vi "Leaktest DAQ v33w.vi"() -> ()   [LabVIEW 2020]
uses:
  Leaktest Temp Mode Select Enum.ctl
  System Directory Type.ctl
  Cfg Cluster Typedef.ctl
  ULx Create Channel (AI-Temperature).vi
  ULx Create Channel (DO-Digital Output).vi
  ULx Create Channel (DI-Digital Input).vi
  ULx Read (Analog 1D DBL NChan 1Samp).vi
  ULx Write (Digital 1D Bool 1Chan 1Samp).vi
  ULx Read (Digital 1D Bool 1Chan 1Samp).vi
panel:
  in  "USB Temp mS":u32=5
  in  "Fallback Location":T2={"Log directory type"=1, "Rel Log Path"="LeakTestData"} {"Log directory type" items=["User Home"=0, "User Desktop"=1, "User Documents"=2, "User Application Data"=3, "User Preferences"=4, "User Temporary"=5, "Public Documents"=6, "Public Application Data"=7, "Public Preferences"=8, "Public Cache"=13, "System Core Libraries"=9, "System Installed Libraries"=10, "Application Files"=11, "Boot Volume Root"=12]}
  in  "Log Dir Path":path=path "\\\\spa-mu2e-network\\Files/LeakRateRawData"
  out "TP loop mS":u32(slide) scale=0.0..100.0
  in  "Chart Dly mS":u32=10
  out "Max Chart Hrs":dbl
  out "Actual cfg file path":path
  in  "Save Cfg":bool
  out "Config Clst":T3={"Log Dir Path"=path "\\\\spa-mu2e-network\\Files/LeakRateRawData", "File Log Sec"=30.0, "34970A Sec"=1.0, "Chart hrs1"=0.25, "Chart hrs2"=0.25, "Filnen Fmt"="%y%m%d_%H%M_MN#.txt", "Temp chans"="Dev1/Ti0, Dev1/Ti2, Dev1/Ti4", "DI Lines"="Dev1/AuxPort/Di2:3", "DO Lines"="Dev1/AuxPort/Do0:1", "VISA ID 34970A"="34970A", "Baud Rate"=enum."38400", "Time Fmt"=enum."Days"} {"Chart hrs2" format="%.1f"; "Chart hrs1" format="%.1f"; "34970A Sec" format="%.1f"; "File Log Sec" format="%.1f"}
  in  "Cfg Filename":string="Leaktest.ini"
  in  "Cfg File Loc":T4={"Cfg directory type"=3, "Rel Log Path"="LeakTest"} {"Cfg directory type" items=["User Home"=0, "User Desktop"=1, "User Documents"=2, "User Application Data"=3, "User Preferences"=4, "User Temporary"=5, "Public Documents"=6, "Public Application Data"=7, "Public Preferences"=8, "Public Cache"=13, "System Core Libraries"=9, "System Installed Libraries"=10, "Application Files"=11, "Boot Volume Root"=12]}
  in  "Time Fmt":enum16{"H:M:S", "Days", "Secs"}(ring)=enum."Days"
  in  "Filnename Format":string="%y%m%d_%H%M_MN#.txt"
  in  "File Log Sec":u32=30
  in  "Header":string[](array[string])=["Elap days", "Fill PSIA", "Ref PSIA", "Diff \"H2O", "Encl degC", "Room degC", "Heater %"]
  out "Heat Safety 2":bool
  out "Heat Safety 1":bool
  in  "Chart Hrs 2":dbl=0.5 min=0.25 max=24.0 step=0.25
  in  "Chart t0 Hrs 2":dbl min=0.0 max=23.0 step=0.25
  in  "Chart t0 Hrs 1":dbl min=0.0 max=23.0 step=0.25
  in  "Chart Hrs 1":dbl=0.5 min=0.25 max=24.0 step=0.25
  in  "34970A Scan Sec":u32=10
  in  "Pressures":T5
  in  "Press Scaling":T6(array[cluster])=[{"Gain"=5.0, "Offset"=0.0, "Units"="PSI", "Channel"="101", "Name"="Fill 1"}, {"Gain"=7.5, "Offset"=-7.5, "Units"="PSI", "Channel"="102", "Name"="Ref 1"}, {"Gain"=2.0, "Offset"=0.0, "Units"="H2O", "Channel"="103", "Name"="Diff 1"}, {"Gain"=7.5, "Offset"=-7.5, "Units"="PSI", "Channel"="104", "Name"="Fill 2"}, {"Gain"=7.5, "Offset"=-7.46, "Units"="PSI", "Channel"="105", "Name"="Ref 2"}, {"Gain"=2.0, "Offset"=-0.038, "Units"="H2O", "Channel"="106", "Name"="Diff 2"}]
  in  "VISA 34970A":refnum<visa-resource-name>="34970A"
  in  "34970A RS232 Cfg":T7={"Timeout Value (10000)"=2000, "Baud Rate"=enum."38400", "Flow Control (1:XON / XOFF)"=enum."RTS / CTS"}
  out "Diff H2O 2":dbl format="%.3f"
  out "Heat% 2":dbl
  out "Heat% 1":dbl
  out "Heat% Cht 2":dbl(graph)
  out "Heat% Cht 1":dbl(graph)
  in  "DI Lines":refnum<k21>="Dev1/AuxPort/Di2:3"
  in  "DO Lines":refnum<k21>="Dev1/AuxPort/Do0:1"
  in  "Temp input chans":refnum<k21>="Dev1/Ti0, Dev1/Ti2, Dev1/Ti4"
  in  "TP Cycle  mS":dbl=5000.0 min=1000.0 max=30000.0
  in  "TP loop mS":u32=50
  out "Heater Safety":cluster{"Encl 1":bool, "Encl 2":bool}
  in  "Heater Out  T/F":bool[](array[boolean])
  in  "Temp Intvl Sec":u32=1
  in  "output range":cluster{"output high":dbl, "output low":dbl}={"output high"=100.0, "output low"=0.0}
  in  "Control Params":T8={"Setpt C"=24.0, "PID"={" gain (Kc)"=180.0, "integral min"=5.0, "derivative min"=0.0}} {"Setpt C" format="%.2f"; "PID"."derivative min" format="%.3f"; "PID"."integral min" format="%.3f"; "PID"."gain (Kc)" format="%.3f"}
  out "error out":errorcluster
  in  "Manual %":cluster{"Man 1":dbl, "Man 2":dbl} {"Man 2" format="%.1f"; "Man 1" format="%.1f"}
  in  "Control Mode":cluster{"Encl 1":T9, "Encl 2":T9}
  out "Heat%":dbl[](array[numeric]) format="%.2f"
  out "Exit 2":bool
  out "Filename 2":string
  in  "Test stop 2":bool
  out "Run/Stop 2":bool
  in  "Test start 2":bool
  out "Room degC 2":dbl format="%.2f"
  out "Encl degC 2":dbl format="%.2f"
  out "Absolute Pressure Cht 2":cluster{"Fill PSIA 1":dbl, "Fill PSIA 2":dbl}(graph)
  out "Diff Pressure Cht 2":dbl(graph)
  out "Temperature Cht 2":T10(graph)
  out "Ref PSIA 2":dbl format="%.2f"
  out "Fill PSIA 2":dbl format="%.2f"
  out "Filename 1":string
  in  "Test stop 1":bool
  out "Run/Stop 1":bool
  in  "Test start 1":bool
  out "Room degC 1":dbl format="%.2f"
  out "Encl degC 1":dbl format="%.2f"
  out "Absolute Pressure Cht 1":cluster{"Fill PSIA 1":dbl, "Fill PSIA 2":dbl}(graph)
  out "Diff Pressure Cht 1":dbl(graph)
  out "Temperature Cht 1":T10(graph)
  in  "Exit":bool
  out "Ref PSIA 1":dbl format="%.2f"
  out "Diff H2O  1":dbl format="%.3f"
  out "Fill PSIA 1":dbl format="%.2f"
  # "`"
  # "```"
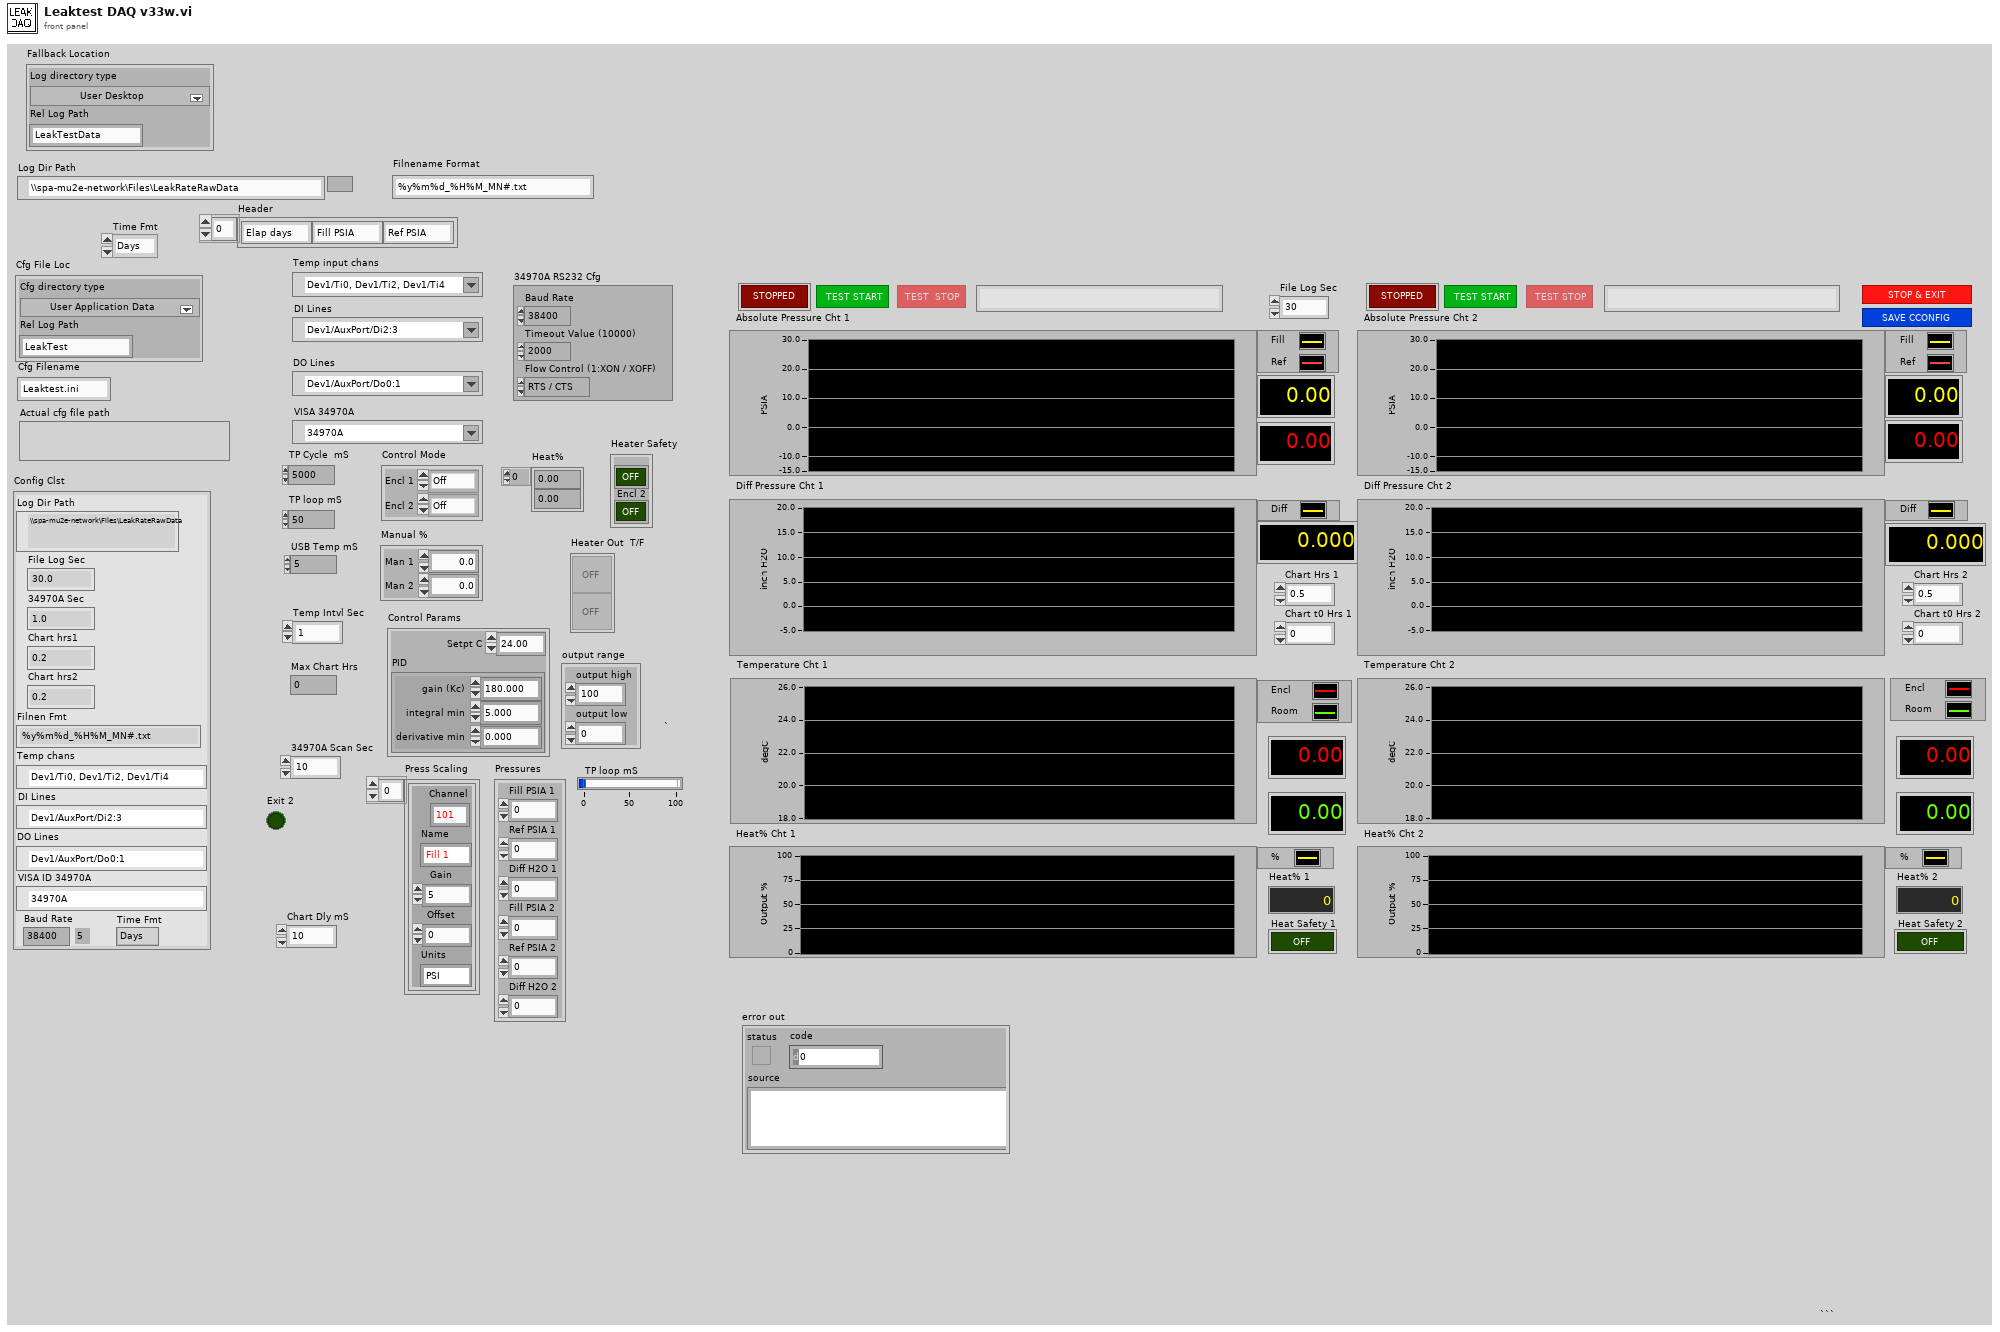
[diagram p1: front panel]
types:
  T1 = typedef "System Directory Type.ctl" = i32
  T2 = cluster{"Log directory type":T1, "Rel Log Path":string}
  T3 = typedef "Cfg Cluster Typedef.ctl" = cluster{"Log Dir Path":path, "File Log Sec":dbl, "34970A Sec":dbl, "Chart hrs1":dbl, "Chart hrs2":dbl, "Filnen Fmt":string, "Temp chans":refnum<k21>, "DI Lines":refnum<k21>, "DO Lines":refnum<k21>, "VISA ID 34970A":refnum<visa-resource-name>, "Baud Rate":enum16{"1200", "2400", "4800", "9600", "19200", "38400", "57600", "115200"}, "Time Fmt":enum16{"H:M:S", "Days", "Secs"}}
  T4 = cluster{"Cfg directory type":T1, "Rel Log Path":string}
  T5 = cluster{"Fill PSIA 1":dbl, "Ref PSIA 1":dbl, "Diff H2O 1":dbl, "Fill PSIA 2":dbl, "Ref PSIA 2":dbl, "Diff H2O 2":dbl}
  T6 = cluster{"Gain":dbl, "Offset":dbl, "Units":string, "Channel":string, "Name":string}[]
  T7 = cluster{"Timeout Value (10000)":u32, "Baud Rate":enum16{"1200", "2400", "4800", "9600", "19200", "38400", "57600", "115200"}, "Flow Control (1:XON / XOFF)":enum16{"None", "XON / XOFF", "RTS / CTS", "DTR / DSR"}}
  T8 = cluster{"Setpt C":dbl, "PID":cluster{" gain (Kc)":dbl, "integral min":dbl, "derivative min":dbl}}
  T9 = typedef "Leaktest Temp Mode Select Enum.ctl" = enum16{"Off", "Manual", "Auto"}
  T10 = cluster{"Temperature 7":dbl, "Temperature 8":dbl}
  T11 = enum16{"Remote Trigger", "Immediate Trigger", "Wait for Trigger", "Abort Scan"}
  T12 = enum8{"Enabled", "Disabled", "Disabled and Grayed Out"}
  T13 = enum16{"1200", "2400", "4800", "9600", "19200", "38400", "57600", "115200"}
  T14 = cluster{"data[0]":dbl, "data[1]":dbl, "data[2]":dbl}
  T15 = cluster{"Fill PSIA 1":dbl, "Ref PSIA 1":dbl, "Diff H2O  1":dbl, "Encl degC 1":dbl, "Room degC 1":dbl, "Heat% 1":dbl}
  T16 = cluster{"Fill PSIA 2":dbl, "Ref PSIA 2":dbl, "Diff H2O 2":dbl, "Encl degC 2":dbl, "Room degC 2":dbl, "Heat% 2":dbl}
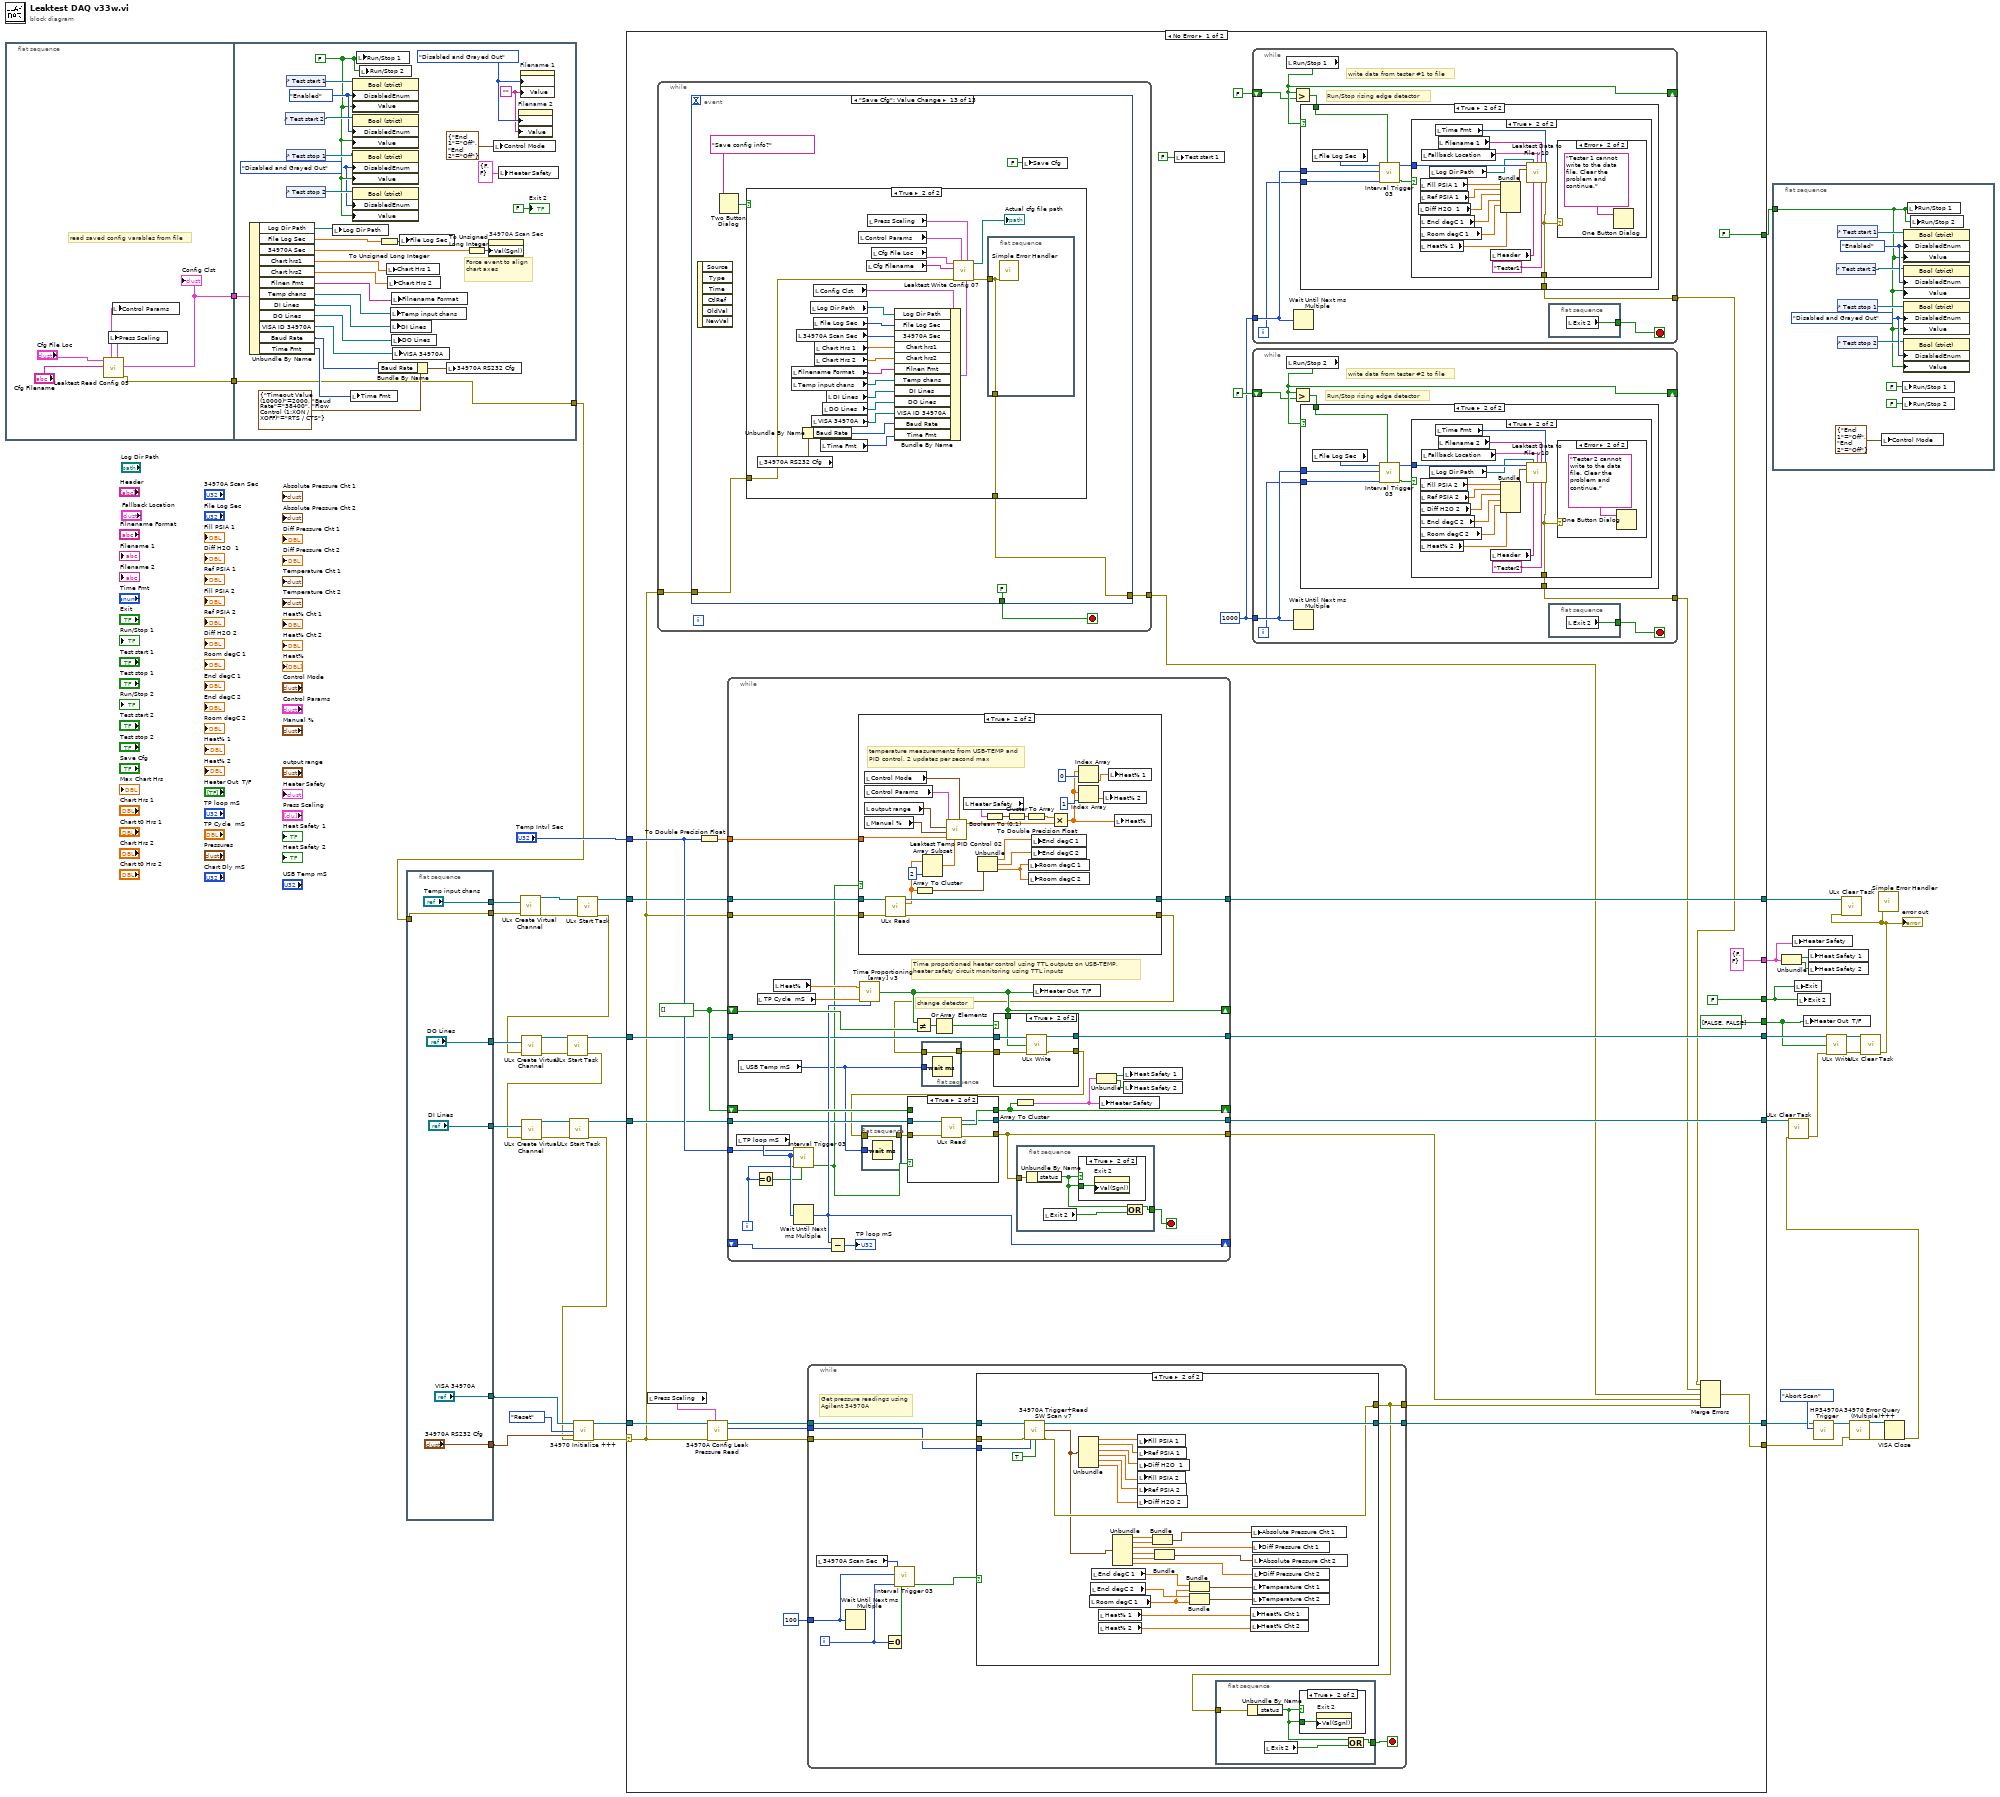
[diagram p0: block diagram]
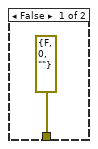
[diagram p2: hidden frame]
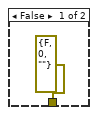
[diagram p3: hidden frame]
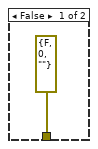
[diagram p7: hidden frame]
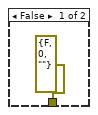
[diagram p8: hidden frame]
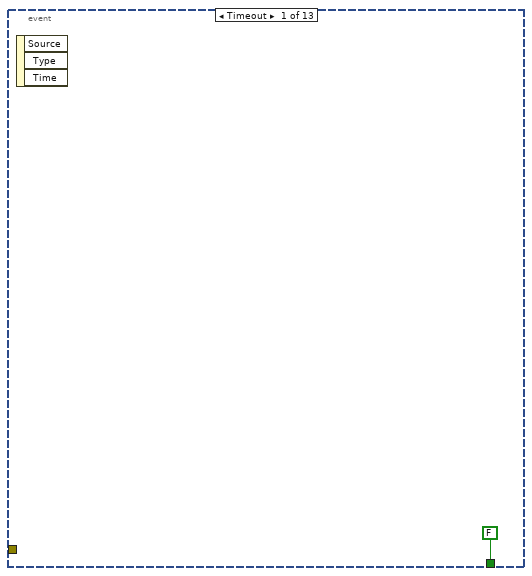
[diagram p10: hidden frame]
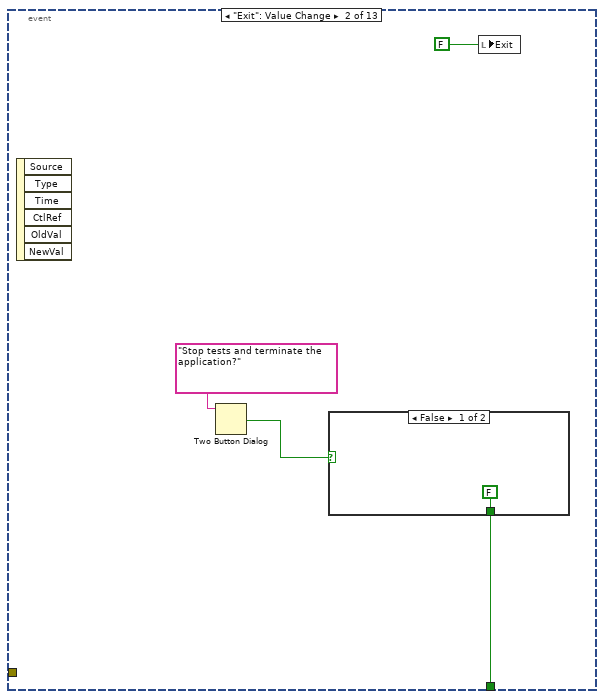
[diagram p11: hidden frame]
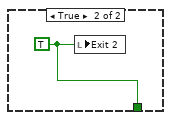
[diagram p12: hidden frame]
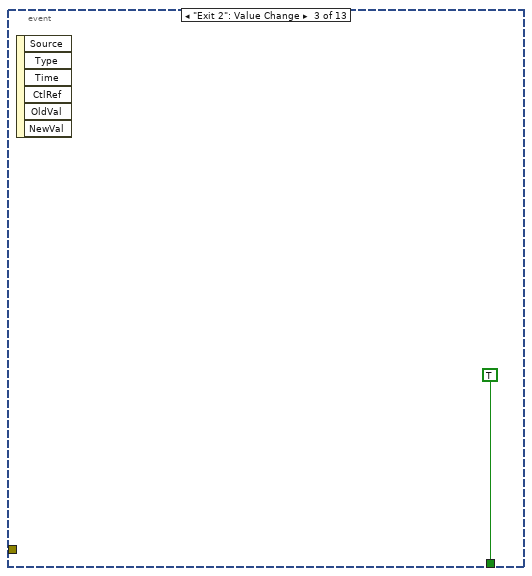
[diagram p13: hidden frame]
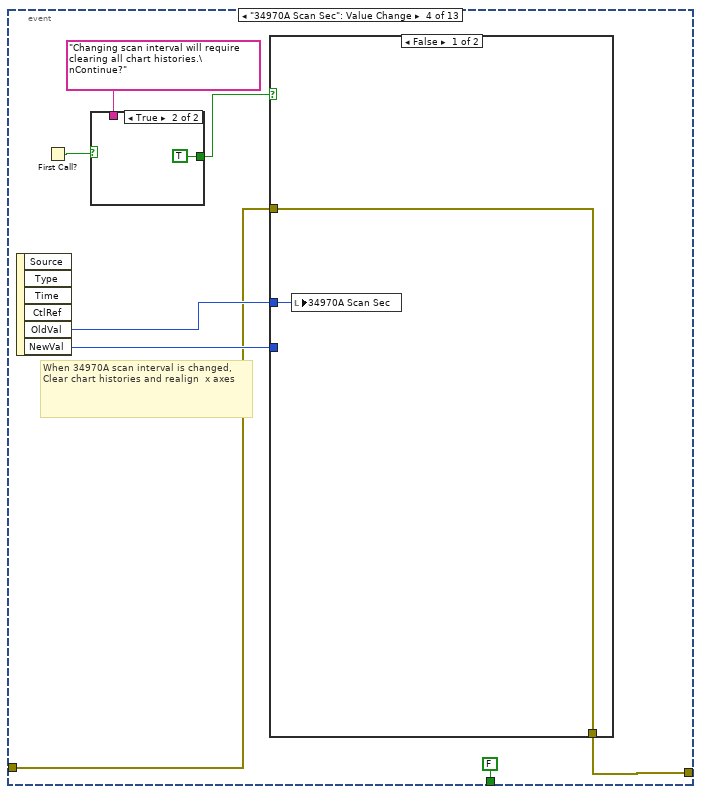
[diagram p14: hidden frame]
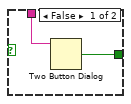
[diagram p15: hidden frame]
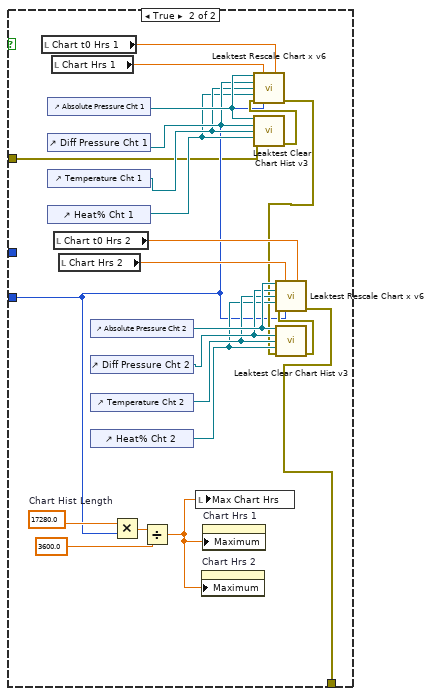
[diagram p16: hidden frame]
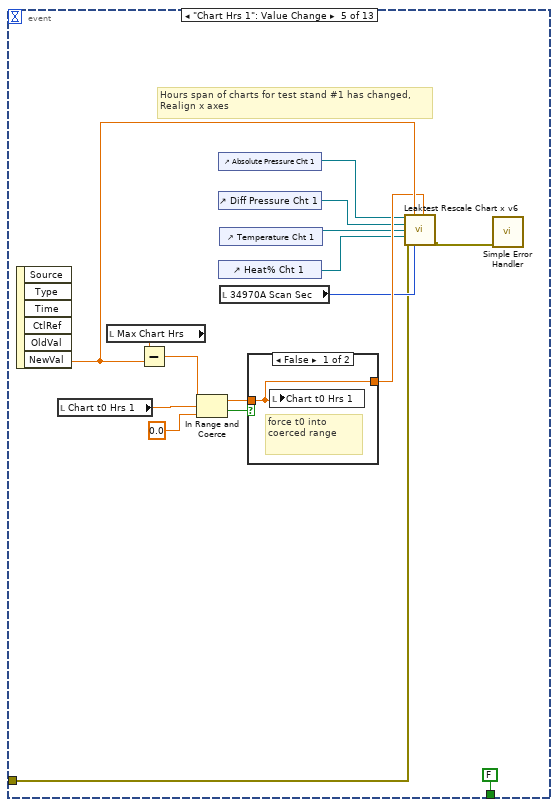
[diagram p17: hidden frame]
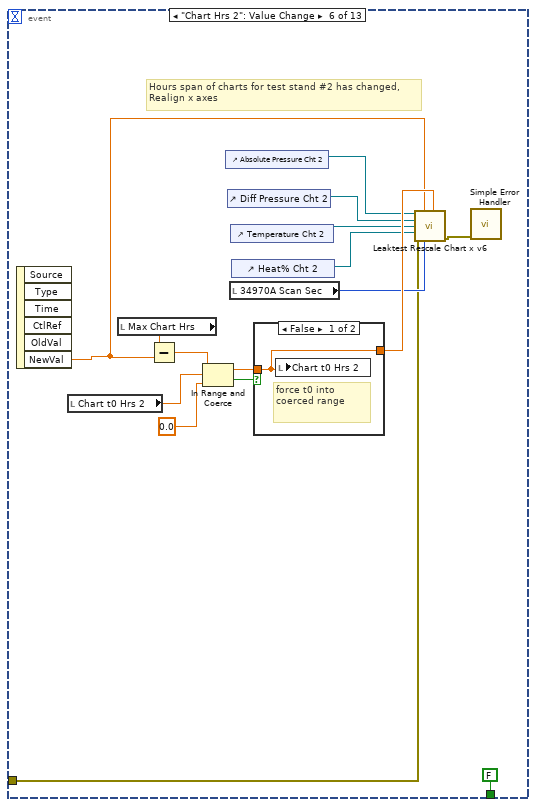
[diagram p19: hidden frame]
diagram:
  n1 = flat-sequence {
    tunnel: [w49] -> w40
    tunnel: [w46] -> w37
    tunnel: [w52] -> w41
    tunnel: w40 -> [w73]
    tunnel: w37 -> [w52]
    frame #0 {
      # "read saved config varables from file"
      n2 = call "Leaktest Read Config 05.vi"("Cfg Filename"="Cfg Filename", "File Location"="Cfg File Loc") -> ("error out"=w46:errorcluster, "Config Clst"=w49:T3, "Press Scaling"=w48:T6, "Control Params"=w47:T8)  [unwired: 3 in, 1 out]
      "Config Clst" <- w49
      n3 = local write "Press Scaling"(w48) -> ()
      n4 = local write "Control Params"(w47) -> ()
    }
    frame #1 {
      w61 = T12."Disabled and Grayed Out" ("Disabled")
      w60 = "" ("Filename 1")
      w74 = T12."Disabled and Grayed Out" ("Disabled")
      w76 = T12."Enabled" ("Disabled")
      w75 = FALSE ("Run/Stop 1")
      # "Force event to align chart axes"
      n5 = Unbundle By Name(w73) -> ("Log Dir Path"=w53:path, "File Log Sec"=w72:dbl, "34970A Sec"=w59:dbl, "Chart hrs1"=w71:dbl, "Chart hrs2"=w70:dbl, "Filnen Fmt"=w69:string, "Temp chans"=w68:refnum<k21>, "DI Lines"=w67:refnum<k21>, "DO Lines"=w66:refnum<k21>, "VISA ID 34970A"=w65:refnum<visa-resource-name>, "Baud Rate"=w63:T13, "Time Fmt"=w62:enum16{"H:M:S", "Days", "Secs"})
      n6 = control-ref of="Test start 2"() -> (w79:refnum<vi>)
      n7 = control-ref of="Test start 1"() -> (w80:refnum<vi>)
      n8 = control-ref of="Test stop 1"() -> (w78:refnum<vi>)
      n9 = control-ref of="Test stop 2"() -> (w77:refnum<vi>)
      n10 = local write "Log Dir Path"(w53) -> ()
      n11 = local write "Time Fmt"(w62) -> ()
      n12 = property class="Bool (strict)"(reference=w80, "DisabledEnum"=w76, "Value"=w75) -> ()  [unwired: 1 in, 2 out]
      n13 = property class="Bool (strict)"(reference=w79, "DisabledEnum"=w76, "Value"=w75) -> ()  [unwired: 1 in, 2 out]
      n14 = property class="Bool (strict)"(reference=w78, "DisabledEnum"=w74, "Value"=w75) -> ()  [unwired: 1 in, 2 out]
      n15 = property class="Bool (strict)"(reference=w77, "DisabledEnum"=w74, "Value"=w75) -> ()  [unwired: 1 in, 2 out]
      n16 = local write "Run/Stop 1"(w75) -> ()
      n17 = local write "Run/Stop 2"(w75) -> ()
      n18 = Bundle By Name(cluster=T7 {"Timeout Value (10000)"=2000, "Baud Rate"=enum."38400", "Flow Control (1:XON / XOFF)"=enum."RTS / CTS"} ("34970A RS232 Cfg"), "Baud Rate"=w63) -> (w64:T7)
      n19 = To Unsigned Long Integer(number=w72) -> (unsigned 32bit integer=w57:u32)
      n20 = local write "Chart Hrs 1"(w71) -> ()
      n21 = local write "Chart Hrs 2"(w70) -> ()
      n22 = local write "Temp input chans"(w68) -> ()
      n23 = local write "DI Lines"(w67) -> ()
      n24 = local write "Filnename Format"(w69) -> ()
      n25 = local write "DO Lines"(w66) -> ()
      n26 = local write "VISA 34970A"(w65) -> ()
      n27 = local write "File Log Sec"(w57) -> ()
      n28 = local write "34970A RS232 Cfg"(w64) -> ()
      n29 = To Unsigned Long Integer(number=w59) -> (unsigned 32bit integer=w58:u32)
      n30 = property on="34970A Scan Sec" class="DigNum (strict)"("Val(Sgnl)"=w58) -> ()  [unwired: 2 in, 2 out]
      n31 = local write "Control Mode"(cluster{"Encl 1":T9, "Encl 2":T9} {"Encl 1"=enum."Off", "Encl 2"=enum."Off"} ("Control Mode")) -> ()
      n32 = local write "Heater Safety"(cluster{"Encl 1":bool, "Encl 2":bool} {"Encl 1"=FALSE, "Encl 2"=FALSE} ("Heater Safety")) -> ()
      n33 = property on="Filename 2" class="Str"("DisabledEnum"=w61, "Value"=w60) -> ()  [unwired: 2 in, 2 out]
      n34 = property on="Filename 1" class="Str"("DisabledEnum"=w61, "Value"=w60) -> ()  [unwired: 2 in, 2 out]
      "Exit 2" <- FALSE ("Exit 2")
    }
  }
  n35 = flat-sequence {
    tunnel: ["Temp input chans"] -> w34
    tunnel: ["DO Lines"] -> w30
    tunnel: ["DI Lines"] -> w26
    tunnel: ["34970A RS232 Cfg"] -> w23
    tunnel: ["VISA 34970A"] -> w24
    tunnel: w41 -> [w82]
    tunnel: [w82] -> w33
    frame #0 {
    }
  }
  n36 = call-poly "ULx Create Virtual Channel.vi"("physical channels"=w34, "error in"=w33) -> ("task out"=w36:refnum<k24>, "error out"=w35:errorcluster)  [unwired: 12 in]
  n37 = call "ULx Start Task.vi"("task in"=w36, "error in"=w35) -> ("task out"=w4:refnum<k24>, "error out"=w29:errorcluster)  [unwired: 12 in]
  n38 = call-poly "ULx Create Virtual Channel.vi"("lines"=w30, "error in"=w29) -> ("task out"=w32:refnum<k24>, "error out"=w31:errorcluster)  [unwired: 12 in]
  n39 = call "ULx Start Task.vi"("task in"=w32, "error in"=w31) -> ("task out"=w6:refnum<k24>, "error out"=w25:errorcluster)  [unwired: 12 in]
  n40 = call-poly "ULx Create Virtual Channel.vi"("lines"=w26, "error in"=w25) -> ("task out"=w28:refnum<k24>, "error out"=w27:errorcluster)  [unwired: 12 in]
  n41 = call "ULx Start Task.vi"("task in"=w28, "error in"=w27) -> ("task out"=w12:refnum<k24>, "error out"=w20:errorcluster)  [unwired: 12 in]
  n42 = call "34970 Initialize +++.vi"("VISA resource name"=w24, "Instr Config"=enum16{"no change", "Reset", "Preset"}."Reset", "Serial Port Configuration"=w23, "error in (no error)"=w20) -> ("VISA session"=w19:refnum<visa-resource-name>, "error out"=w21:errorcluster)  [unwired: 10 in]
  n43 = case shown="No Error" w21 {
    selector: w21 -> [w89 w550]
    tunnel: "Temp Intvl Sec" -> [w113 _]
    tunnel: [FALSE ("Exit 2") FALSE ("Exit 2")] -> w39
    tunnel: [w88 w550] -> w14
    tunnel: [cluster{"Encl 1":bool, "Encl 2":bool} {"Encl 1"=FALSE, "Encl 2"=FALSE} ("Heater \nSafety") cluster{"Encl 1":bool, "Encl 2":bool} {"Encl 1"=FALSE, "Encl 2"=FALSE} ("Heater \nSafety")] -> w42
    tunnel: [bool[] [FALSE, FALSE] ("data") bool[] [FALSE, FALSE] ("data")] -> w1
    tunnel: [FALSE ("Run/Stop 1") FALSE ("Run/Stop 1")] -> w38
    tunnel: w19 -> [w109 w543]
    tunnel: [w106 w543] -> w13
    tunnel: w12 -> [w105 w544]
    tunnel: [w104 w544] -> w9
    tunnel: w6 -> [w103 w545]
    tunnel: [w102 w545] -> w5
    tunnel: w4 -> [w101 w546]
    tunnel: [w99 w546] -> w3
    frame No Error {
      w92 = u32 1000 ("Loop mS")
      w118 = bool[] [] ("Relay Output")
      n44 = local read "Press Scaling"() -> (w95:T6)
      n45 = while {
        tunnel: [w232] -> w97
        tunnel: w89 -> [w231]
        stop <- w233 stop-if-true
        n46 = event shown="[12] \"Save Cfg\": Value Change" {
          selector: _ -> [_ _ _ _ _ _ _ _ _ _ _ _ _]
          dyn-events: _ -> [_ _ _ _ _ _ _ _ _ _ _ _ _]
          timeout: _ -> [_ _ _ _ _ _ _ _ _ _ _ _ _]
          tunnel: [FALSE ("Exit 2") w238 TRUE ("Exit 2") FALSE ("Exit 2") FALSE ("Exit 2") FALSE ("Exit 2") FALSE ("Exit 2") FALSE ("Exit 2") _ FALSE ("Exit 2") _ _ FALSE ("Exit 2")] -> w233
          tunnel: [_ _ _ w243 _ _ _ _ _ _ _ _ w428] -> w232
          tunnel: w231 -> [_ _ _ w242 w277 w295 w313 w331 _ _ _ _ w426]
          event Timeout {
            n47 = event-data() -> ()  [unwired: 1 in, 3 out]
          }
          event "Exit": Value Change {
            n48 = event-data() -> ()  [unwired: 1 in, 6 out]
            n49 = Two Button Dialog(message="Stop tests and terminate the application?") -> (T button?=w236:bool)  [unwired: 2 in]
            n50 = case shown="False" w236 {
              tunnel: [FALSE ("Exit 2") w240] -> w238
              frame False {
              }
              frame True {
                w240 = TRUE ("Exit 2")
                n51 = local write "Exit 2"(w240) -> ()
              }
            }
            n52 = local write "Exit"(FALSE ("Run/Stop 1")) -> ()
          }
          event "Exit 2": Value Change {
            n53 = event-data() -> ()  [unwired: 1 in, 6 out]
          }
          event "34970A Scan Sec": Value Change {
            # "When 34970A scan interval is changed, Clear chart histories and realign  x axes"
            n54 = event-data() -> ("OldVal"=w247:u32, "NewVal"=w244:u32)  [unwired: 1 in, 4 out]
            n55 = First Call?() -> (First Call?: T/F=w246:bool)
            n56 = case shown="True" w246 {
              tunnel: "Changing scan interval will require clearing all chart histories.\nContinue?" ("message") -> [w251 _]
              tunnel: [w250 TRUE ("T button?")] -> w245
              frame False {
                n57 = Two Button Dialog(message=w251) -> (T button?=w250:bool)  [unwired: 2 in]
              }
              frame True {
              }
            }
            n58 = case shown="False" w245 {
              tunnel: w244 -> [_ w256]
              tunnel: w247 -> [w254 _]
              tunnel: [w253 w257] -> w243
              tunnel: w242 -> [w253 w255]
              frame False {
                n59 = local write "34970A Scan Sec"(w254) -> ()
              }
              frame True {
                w264 = 17280.0  # Chart Hist Length
                n60 = local read "Chart t0 Hrs 1"() -> (w268:dbl)
                n61 = control-ref of="Absolute Pressure Cht 1"() -> (w276:refnum<vi>)
                n62 = control-ref of="Diff Pressure Cht 1"() -> (w275:refnum<vi>)
                n63 = control-ref of="Temperature Cht 1"() -> (w274:refnum<vi>)
                n64 = control-ref of="Heat% Cht 1"() -> (w273:refnum<vi>)
                n65 = local read "Chart Hrs 1"() -> (w267:dbl)
                n66 = local read "Chart t0 Hrs 2"() -> (w266:dbl)
                n67 = local read "Chart Hrs 2"() -> (w265:dbl)
                n68 = control-ref of="Absolute Pressure Cht 2"() -> (w272:refnum<vi>)
                n69 = control-ref of="Diff Pressure Cht 2"() -> (w271:refnum<vi>)
                n70 = control-ref of="Temperature Cht 2"() -> (w270:refnum<vi>)
                n71 = control-ref of="Heat% Cht 2"() -> (w269:refnum<vi>)
                n72 = Multiply(x=w264, y=w256) -> (x*y=w263:dbl)
                n73 = Divide(x=w263, y=3600.0) -> (x/y=w261:dbl)
                n74 = local write "Max Chart Hrs"(w261) -> ()
                n75 = property on="Chart Hrs 2" class="DigNum (strict)"("Maximum"=w261) -> ()  [unwired: 2 in, 2 out]
                n76 = property on="Chart Hrs 1" class="DigNum (strict)"("Maximum"=w261) -> ()  [unwired: 2 in, 2 out]
                n77 = call "Leaktest Clear Chart Hist v3.vi"("Absolute Pres Cht Ref"=w276, "Diff Pres Cht Ref"=w275, "Temp Cht Ref"=w274, "Heat % Cht ref"=w273, "error in (no error)"=w255) -> ("error out"=w260:errorcluster)  [unwired: 10 in]
                n78 = call "Leaktest Rescale Chart x v6.vi"("Absolute Pres Cht Ref"=w276, "Chart Hrs"=w267, "Chart Zero"=w268, "Diff Pres Cht Ref"=w275, "Temp Cht Ref"=w274, "Heat % Cht ref"=w273, "error in (no error)"=w260, "X Mult sec"=w256) -> ("error out"=w259:errorcluster)  [unwired: 7 in]
                n79 = call "Leaktest Clear Chart Hist v3.vi"("Absolute Pres Cht Ref"=w272, "Diff Pres Cht Ref"=w271, "Temp Cht Ref"=w270, "Heat % Cht ref"=w269, "error in (no error)"=w259) -> ("error out"=w258:errorcluster)  [unwired: 10 in]
                n80 = call "Leaktest Rescale Chart x v6.vi"("Absolute Pres Cht Ref"=w272, "Chart Hrs"=w265, "Chart Zero"=w266, "Diff Pres Cht Ref"=w271, "Temp Cht Ref"=w270, "Heat % Cht ref"=w269, "error in (no error)"=w258, "X Mult sec"=w256) -> ("error out"=w257:errorcluster)  [unwired: 7 in]
              }
            }
          }
          event "Chart Hrs 1": Value Change {
            # "Hours span of charts for test stand #1 has changed,\nRealign x axes"
            n81 = event-data() -> ("NewVal"=w287:dbl)  [unwired: 1 in, 5 out]
            n82 = local read "Chart t0 Hrs 1"() -> (w290:dbl)
            n83 = local read "Max Chart Hrs"() -> (w279:dbl)
            n84 = Subtract(x=w279, y=w287) -> (x-y=w292:dbl)
            n85 = In Range and Coerce(upper limit=w292, x=w290, lower limit=0.0) -> (coerced(x)=w288:dbl, In Range?=w289:bool)
            n86 = control-ref of="Absolute Pressure Cht 1"() -> (w281:refnum<vi>)
            n87 = control-ref of="Diff Pressure Cht 1"() -> (w284:refnum<vi>)
            n88 = control-ref of="Heat% Cht 1"() -> (w282:refnum<vi>)
            n89 = control-ref of="Temperature Cht 1"() -> (w283:refnum<vi>)
            n90 = local read "34970A Scan Sec"() -> (w285:u32)
            n91 = case shown="False" w289 {
              tunnel: w288 -> [w293 w294]
              tunnel: [w293 w294] -> w286
              frame False {
                # "force t0 into coerced range"
                n92 = local write "Chart t0 Hrs 1"(w293) -> ()
              }
              frame True {
              }
            }
            n93 = call "Leaktest Rescale Chart x v6.vi"("Absolute Pres Cht Ref"=w281, "Chart Hrs"=w287, "Chart Zero"=w286, "Diff Pres Cht Ref"=w284, "Temp Cht Ref"=w283, "Heat % Cht ref"=w282, "error in (no error)"=w277, "X Mult sec"=w285) -> ("error out"=w278:errorcluster)  [unwired: 7 in]
            n94 = call "Simple Error Handler.vi"("error in (no error)"=w278) -> ()  [unwired: 4 in, 5 out]
          }
          event "Chart Hrs 2": Value Change {
            # "Hours span of charts for test stand #2 has changed,\nRealign x axes"
            n95 = event-data() -> ("NewVal"=w303:dbl)  [unwired: 1 in, 5 out]
            n96 = local read "Chart t0 Hrs 2"() -> (w309:dbl)
            n97 = local read "Max Chart Hrs"() -> (w297:dbl)
            n98 = Subtract(x=w297, y=w303) -> (x-y=w310:dbl)
            n99 = In Range and Coerce(upper limit=w310, x=w309, lower limit=0.0) -> (coerced(x)=w307:dbl, In Range?=w308:bool)
            n100 = control-ref of="Absolute Pressure Cht 2"() -> (w299:refnum<vi>)
            n101 = control-ref of="Diff Pressure Cht 2"() -> (w300:refnum<vi>)
            n102 = local read "34970A Scan Sec"() -> (w305:u32)
            n103 = control-ref of="Temperature Cht 2"() -> (w301:refnum<vi>)
            n104 = control-ref of="Heat% Cht 2"() -> (w302:refnum<vi>)
            n105 = case shown="False" w308 {
              tunnel: w307 -> [w311 w312]
              tunnel: [w311 w312] -> w306
              frame False {
                # "force t0 into coerced range"
                n106 = local write "Chart t0 Hrs 2"(w311) -> ()
              }
              frame True {
              }
            }
            n107 = call "Leaktest Rescale Chart x v6.vi"("Absolute Pres Cht Ref"=w299, "Chart Hrs"=w303, "Chart Zero"=w306, "Diff Pres Cht Ref"=w300, "Temp Cht Ref"=w301, "Heat % Cht ref"=w302, "error in (no error)"=w295, "X Mult sec"=w305) -> ("error out"=w296:errorcluster)  [unwired: 7 in]
            n108 = call "Simple Error Handler.vi"("error in (no error)"=w296) -> ()  [unwired: 4 in, 5 out]
          }
          event "Chart t0 Hrs 1": Value Change {
            # "t-zero of charts for test stand #1 has changed,\nRealign x axes"
            n109 = event-data() -> ("NewVal"=w324:dbl)  [unwired: 1 in, 5 out]
            n110 = local read "Max Chart Hrs"() -> (w315:dbl)
            n111 = local read "Chart Hrs 1"() -> (w317:dbl)
            n112 = Subtract(x=w315, y=w317) -> (x-y=w328:dbl)
            n113 = In Range and Coerce(upper limit=w328, x=w324, lower limit=0.0) -> (coerced(x)=w326:dbl, In Range?=w327:bool)
            n114 = control-ref of="Absolute Pressure Cht 1"() -> (w319:refnum<vi>)
            n115 = control-ref of="Diff Pressure Cht 1"() -> (w322:refnum<vi>)
            n116 = control-ref of="Heat% Cht 1"() -> (w320:refnum<vi>)
            n117 = control-ref of="Temperature Cht 1"() -> (w321:refnum<vi>)
            n118 = local read "34970A Scan Sec"() -> (w323:u32)
            n119 = case shown="False" w327 {
              tunnel: w326 -> [w329 w330]
              tunnel: [w329 w330] -> w318
              frame False {
                # "force t0 into coerced range"
                n120 = local write "Chart t0 Hrs 1"(w329) -> ()
              }
              frame True {
              }
            }
            n121 = call "Leaktest Rescale Chart x v6.vi"("Absolute Pres Cht Ref"=w319, "Chart Hrs"=w317, "Chart Zero"=w318, "Diff Pres Cht Ref"=w322, "Temp Cht Ref"=w321, "Heat % Cht ref"=w320, "error in (no error)"=w313, "X Mult sec"=w323) -> ("error out"=w314:errorcluster)  [unwired: 7 in]
            n122 = call "Simple Error Handler.vi"("error in (no error)"=w314) -> ()  [unwired: 4 in, 5 out]
          }
          event "Chart t0 Hrs 2": Value Change {
            # "Hours span of charts for test stand #2 has changed,\nRealign x axes"
            n123 = event-data() -> ("NewVal"=w340:dbl)  [unwired: 1 in, 5 out]
            n124 = local read "Max Chart Hrs"() -> (w333:dbl)
            n125 = local read "Chart Hrs 2"() -> (w342:dbl)
            n126 = Subtract(x=w333, y=w342) -> (x-y=w346:dbl)
            n127 = In Range and Coerce(upper limit=w346, x=w340, lower limit=0.0) -> (coerced(x)=w344:dbl, In Range?=w345:bool)
            n128 = control-ref of="Absolute Pressure Cht 2"() -> (w338:refnum<vi>)
            n129 = control-ref of="Diff Pressure Cht 2"() -> (w337:refnum<vi>)
            n130 = local read "34970A Scan Sec"() -> (w343:u32)
            n131 = control-ref of="Temperature Cht 2"() -> (w336:refnum<vi>)
            n132 = control-ref of="Heat% Cht 2"() -> (w335:refnum<vi>)
            n133 = case shown="False" w345 {
              tunnel: w344 -> [w347 w348]
              tunnel: [w347 w348] -> w339
              frame False {
                # "force t0 into coerced range"
                n134 = local write "Chart t0 Hrs 2"(w347) -> ()
              }
              frame True {
              }
            }
            n135 = call "Leaktest Rescale Chart x v6.vi"("Absolute Pres Cht Ref"=w338, "Chart Hrs"=w342, "Chart Zero"=w339, "Diff Pres Cht Ref"=w337, "Temp Cht Ref"=w336, "Heat % Cht ref"=w335, "error in (no error)"=w331, "X Mult sec"=w343) -> ("error out"=w332:errorcluster)  [unwired: 7 in]
            n136 = call "Simple Error Handler.vi"("error in (no error)"=w332) -> ()  [unwired: 4 in, 5 out]
          }
          event "Test start 1": Value Change {
            # "test stand #1 started"
            # "prevent run/stop from going true until Mod# dialog completes and filename is ready"
            n137 = event-data() -> ("CtlRef"=w371:refnum<vi>)  [unwired: 1 in, 3 out]
            n138 = local read "Filnename Format"() -> (w354:string)
            n139 = local read "Control Mode"() -> (w363:cluster{"Encl 1":T9, "Encl 2":T9})
            n140 = Get Date/Time In Seconds() -> (seconds since 1Jan1904=w359:timestamp)
            n141 = control-ref of="Absolute Pressure Cht 1"() -> (w366:refnum<vi>)
            n142 = control-ref of="Diff Pressure Cht 1"() -> (w369:refnum<vi>)
            n143 = control-ref of="Heat% Cht 1"() -> (w367:refnum<vi>)
            n144 = control-ref of="Temperature Cht 1"() -> (w368:refnum<vi>)
            n145 = control-ref of="Test stop 1"() -> (w364:refnum<vi>)
            n146 = Format Date/Time String(time format string (%c)=w354, seconds (now)=w359) -> (date/time string=w358:string)  [unwired: 1 in]
            n147 = call "Prompt User for Input"("Enable"=TRUE) -> ("Module ID"=w353:string)  [unwired: 16 in, 2 out]
            n148 = Bundle By Name(cluster=w363, "Encl 1"=Leaktest_Temp_Mode_Select_Enum."Auto" ("Pos'n 1")) -> (w362:cluster{"Encl 1":T9, "Encl 2":T9})
            n149 = property class="Bool (strict)"(reference=w364, "DisabledEnum"=T12."Enabled" ("Disabled")) -> ()  [unwired: 1 in, 2 out]
            n150 = property class="Bool (strict)"(reference=w371, "DisabledEnum"=T12."Disabled and Grayed Out" ("Disabled")) -> ()  [unwired: 1 in, 2 out]
            n151 = local write "Control Mode"(w362) -> ()
            n152 = Match Pattern(string=w358, regular expression="#") -> (before substring=w356:string, after substring=w355:string)  [unwired: 1 in, 2 out]
            n153 = call "Leaktest Clear Chart Hist v3.vi"("Absolute Pres Cht Ref"=w366, "Diff Pres Cht Ref"=w369, "Temp Cht Ref"=w368, "Heat % Cht ref"=w367) -> ()  [unwired: 11 in, 1 out]
            n154 = Concatenate Strings(w356, w353, w355) -> (w352:string)
            n155 = flat-sequence {
              tunnel: w352 -> [w373]
              tunnel: [TRUE ("Run/Stop 1")] -> w351
              tunnel: T12."Disabled" ("Disabled") -> [w372]
              frame #0 {
                n156 = property on="Filename 1" class="Str"("DisabledEnum"=w372, "Value"=w373) -> ()  [unwired: 2 in, 2 out]
              }
            }
            n157 = local write "Test start 1"(FALSE ("Run/Stop 1")) -> ()
            n158 = local write "Run/Stop 1"(w351) -> ()
          }
          event "Test stop 1": Value Change {
            n159 = event-data() -> ("CtlRef"=w379:refnum<vi>)  [unwired: 1 in, 3 out]
            n160 = Two Button Dialog(message="Sure you want to stop  Tester1 and close the data file?") -> (T button?=w376:bool)  [unwired: 2 in]
            n161 = case shown="True" w376 {
              tunnel: w379 -> [_ w387]
              frame False {
              }
              frame True {
                w380 = T12."Disabled and Grayed Out" ("Disabled")
                n162 = local read "Control Mode"() -> (w383:cluster{"Encl 1":T9, "Encl 2":T9})
                n163 = control-ref of="Test start 1"() -> (w386:refnum<vi>)
                n164 = local write "Run/Stop 1"(FALSE ("Run/Stop 1")) -> ()
                n165 = Bundle By Name(cluster=w383, "Encl 1"=Leaktest_Temp_Mode_Select_Enum."Off" ("Pos'n 1")) -> (w382:cluster{"Encl 1":T9, "Encl 2":T9})
                n166 = property class="Bool (strict)"(reference=w387, "DisabledEnum"=w380) -> ()  [unwired: 1 in, 2 out]
                n167 = property class="Bool (strict)"(reference=w386, "DisabledEnum"=T12."Enabled" ("Disabled")) -> ()  [unwired: 1 in, 2 out]
                n168 = local write "Control Mode"(w382) -> ()
                n169 = property on="Filename 1" class="Str"("DisabledEnum"=w380) -> ()  [unwired: 2 in, 2 out]
              }
            }
            n170 = local write "Test stop 1"(FALSE ("Run/Stop 1")) -> ()
          }
          event "Test start 2": Value Change {
            # "test stand #2 started"
            # "prevent run/stop from going true until Mod# dialog completes and filename is ready"
            n171 = event-data() -> ("CtlRef"=w409:refnum<vi>)  [unwired: 1 in, 3 out]
            n172 = local read "Filnename Format"() -> (w392:string)
            n173 = control-ref of="Absolute Pressure Cht 2"() -> (w406:refnum<vi>)
            n174 = Get Date/Time In Seconds() -> (seconds since 1Jan1904=w397:timestamp)
            n175 = control-ref of="Diff Pressure Cht 2"() -> (w405:refnum<vi>)
            n176 = control-ref of="Heat% Cht 2"() -> (w403:refnum<vi>)
            n177 = control-ref of="Temperature Cht 2"() -> (w404:refnum<vi>)
            n178 = local read "Control Mode"() -> (w401:cluster{"Encl 1":T9, "Encl 2":T9})
            n179 = control-ref of="Test stop 2"() -> (w407:refnum<vi>)
            n180 = Format Date/Time String(time format string (%c)=w392, seconds (now)=w397) -> (date/time string=w396:string)  [unwired: 1 in]
            n181 = call "Prompt User for Input2"("Enable"=TRUE) -> ("Module ID"=w391:string)  [unwired: 16 in, 2 out]
            n182 = Bundle By Name(cluster=w401, "Encl 2"=Leaktest_Temp_Mode_Select_Enum."Auto" ("Pos'n 1")) -> (w400:cluster{"Encl 1":T9, "Encl 2":T9})
            n183 = property class="Bool (strict)"(reference=w407, "DisabledEnum"=T12."Enabled" ("Disabled")) -> ()  [unwired: 1 in, 2 out]
            n184 = property class="Bool (strict)"(reference=w409, "DisabledEnum"=T12."Disabled and Grayed Out" ("Disabled")) -> ()  [unwired: 1 in, 2 out]
            n185 = Match Pattern(string=w396, regular expression="#") -> (before substring=w394:string, after substring=w393:string)  [unwired: 1 in, 2 out]
            n186 = local write "Control Mode"(w400) -> ()
            n187 = call "Leaktest Clear Chart Hist v3.vi"("Absolute Pres Cht Ref"=w406, "Diff Pres Cht Ref"=w405, "Temp Cht Ref"=w404, "Heat % Cht ref"=w403) -> ()  [unwired: 11 in, 1 out]
            n188 = Concatenate Strings(w394, w391, w393) -> (w390:string)
            n189 = flat-sequence {
              tunnel: [TRUE ("Run/Stop 1")] -> w402
              tunnel: w390 -> [w412]
              tunnel: T12."Disabled" ("Disabled") -> [w411]
              frame #0 {
                n190 = property on="Filename 2" class="Str"("DisabledEnum"=w411, "Value"=w412) -> ()  [unwired: 2 in, 2 out]
              }
            }
            n191 = local write "Run/Stop 2"(w402) -> ()
            n192 = local write "Test start 2"(FALSE ("Run/Stop 1")) -> ()
          }
          event "Test stop 2": Value Change {
            n193 = event-data() -> ("CtlRef"=w417:refnum<vi>)  [unwired: 1 in, 3 out]
            n194 = Two Button Dialog(message="Sure you want to stop Tester2 and close the data file?") -> (T button?=w415:bool)  [unwired: 2 in]
            n195 = case shown="True" w415 {
              tunnel: w417 -> [_ w424]
              frame False {
              }
              frame True {
                w418 = T12."Disabled and Grayed Out" ("Disabled")
                n196 = local read "Control Mode"() -> (w421:cluster{"Encl 1":T9, "Encl 2":T9})
                n197 = control-ref of="Test start 2"() -> (w422:refnum<vi>)
                n198 = local write "Run/Stop 2"(FALSE ("Run/Stop 1")) -> ()
                n199 = Bundle By Name(cluster=w421, "Encl 2"=Leaktest_Temp_Mode_Select_Enum."Off" ("Pos'n 1")) -> (w420:cluster{"Encl 1":T9, "Encl 2":T9})
                n200 = property class="Bool (strict)"(reference=w424, "DisabledEnum"=w418) -> ()  [unwired: 1 in, 2 out]
                n201 = property class="Bool (strict)"(reference=w422, "DisabledEnum"=T12."Enabled" ("Disabled")) -> ()  [unwired: 1 in, 2 out]
                n202 = local write "Control Mode"(w420) -> ()
                n203 = property on="Filename 2" class="Str"("DisabledEnum"=w418) -> ()  [unwired: 2 in, 2 out]
              }
            }
            n204 = local write "Test stop 2"(FALSE ("Run/Stop 1")) -> ()
          }
          event "Save Cfg": Value Change {
            n205 = event-data() -> ()  [unwired: 1 in, 6 out]
            n206 = Two Button Dialog(message="Save config info?") -> (T button?=w429:bool)  [unwired: 2 in]
            n207 = case shown="True" w429 {
              tunnel: [w432 w434] -> w428
              tunnel: w426 -> [w432 w433]
              frame False {
              }
              frame True {
                n208 = local read "34970A RS232 Cfg"() -> (w450:T7)
                n209 = local read "Filnename Format"() -> (w447:string)
                n210 = local read "Temp input chans"() -> (w454:refnum<k21>)
                n211 = local read "34970A Scan Sec"() -> (w444:u32)
                n212 = Unbundle By Name(w450) -> ("Baud Rate"=w449:T13)
                n213 = local read "Log Dir Path"() -> (w435:path)
                n214 = local read "VISA 34970A"() -> (w451:refnum<visa-resource-name>)
                n215 = local read "File Log Sec"() -> (w443:u32)
                n216 = local read "Config Clst"() -> (w455:T3)
                n217 = local read "Chart Hrs 1"() -> (w445:dbl)
                n218 = local read "Chart Hrs 2"() -> (w446:dbl)
                n219 = local read "Time Fmt"() -> (w448:enum16{"H:M:S", "Days", "Secs"})
                n220 = local read "DO Lines"() -> (w452:refnum<k21>)
                n221 = local read "DI Lines"() -> (w453:refnum<k21>)
                n222 = local read "Control Params"() -> (w440:T8)
                n223 = local read "Cfg Filename"() -> (w441:string)
                n224 = local read "Press Scaling"() -> (w439:T6)
                n225 = local read "Cfg File Loc"() -> (w442:T4)
                n226 = Bundle By Name(cluster=w455, "Log Dir Path"=w435, "File Log Sec"=w443, "34970A Sec"=w444, "Chart hrs1"=w445, "Chart hrs2"=w446, "Filnen Fmt"=w447, "Temp chans"=w454, "DI Lines"=w453, "DO Lines"=w452, "VISA ID 34970A"=w451, "Baud Rate"=w449, "Time Fmt"=w448) -> (w438:T3)
                n227 = call "Leaktest Write Config 07.vi"("Config Clst"=w438, "Press Scaling"=w439, "Control Params"=w440, "error in (no error)"=w433, "Cfg Filename"=w441, "Cfg File Location"=w442) -> ("error out"=w437:errorcluster, "Actual file path"=→"Actual cfg file path":path)  [unwired: 4 in]
                n228 = flat-sequence {
                  tunnel: w437 -> [w456]
                  tunnel: [w456] -> w434
                  frame #0 {
                    n229 = call "Simple Error Handler.vi"("error in (no error)"=w456) -> ()  [unwired: 4 in, 5 out]
                  }
                }
              }
            }
            n230 = local write "Save Cfg"(FALSE ("Save Cfg")) -> ()
          }
        }
      }
      n231 = To Double Precision Float(number=w113) -> (double precision float=w114:dbl)
      n232 = call "34970A Config Leak Pressure Read.vi"("Press Scaling"=w95, "error in"=w89, "VISA session"=w109) -> ("error out"=w107:errorcluster, "#channels"=w96:i32, "VISA resource name out"=w108:refnum<visa-resource-name>)  [unwired: 4 in]
      n233 = while {
        shift-right: [w490] -> _
        shift-left: w118 -> [w489]
        shift-right: [w487] -> _
        shift-left: w118 -> [w486]
        tunnel: w114 -> [w479]
        tunnel: w113 -> [w477]
        shift-right: [w473] -> _
        shift-left: _ -> [w474]
        tunnel: w105 -> [w471]
        tunnel: [w470] -> w104
        tunnel: w103 -> [w469]
        tunnel: [w468] -> w102
        tunnel: w101 -> [w467]
        tunnel: [w466] -> w99
        tunnel: w89 -> [w463]
        tunnel: [w462] -> w90
        i -> [w476]
        stop <- w484 stop-if-true
        # "change detector"
        # "Time proportioned heater control using TTL outputs on USB-TEMP,\nheater safety circuit monitoring using TTL inputs"
        n234 = local read "TP loop mS"() -> (w478:u32)
        n235 = local read "USB Temp mS"() -> (w457:u32)
        n236 = Equal To 0?(x=w476) -> (x = 0?=w475:bool)
        n237 = local read "TP Cycle  mS"() -> (w480:dbl)
        n238 = local read "Heat%"() -> (w485:dbl[])
        n239 = Wait Until Next ms Multiple(millisecond multiple=w478) -> (millisecond timer value=w473:u32)
        n240 = call "Interval Trigger 03.vi"("First Call?: T/F"=w475, "Iteration#"=w476, "Loop mS"=w478, "Interval Sec"=w477) -> ("Go"=w464:bool)  [unwired: 3 in, 2 out]
        n241 = Subtract(x=w473, y=w474) -> (x-y=→"TP loop mS":u32)
        n242 = case shown="True" w464 {
          tunnel: w479 -> [_ w522]
          tunnel: [w495 w504] -> w461
          tunnel: w467 -> [w496 w503]
          tunnel: [w496 w502] -> w466
          tunnel: w463 -> [w495 w497]
          frame False {
          }
          frame True {
            # "temperature measurements from USB-TEMP and PID control, 2 updates per second max"
            n243 = local read "Control Mode"() -> (w521:cluster{"Encl 1":T9, "Encl 2":T9})
            n244 = local read "Control Params"() -> (w520:T8)
            n245 = local read "output range"() -> (w519:cluster{"output high":dbl, "output low":dbl})
            n246 = local read "Manual %"() -> (w518:cluster{"Man 1":dbl, "Man 2":dbl})
            n247 = call-poly "ULx Read.vi"("task in"=w503, "error in"=w497) -> ("task out"=w502:refnum<k24>, "data"=w500:dbl[], "error out"=w504:errorcluster)  [unwired: 11 in]
            n248 = Array To Cluster(array=w500) -> (cluster=w498:T14)
            n249 = Array Subset(array=w500, length=2) -> (w499:dbl[])  [unwired: 1 in]
            n250 = call "Leaktest Temp PID Control 02.vi"("Control Mode"=w521, "process variable"=w499, "dt (s)"=w522, "Manual %"=w518, "output range"=w519, "Control Params"=w520) -> ("Output %"=w509:dbl[])  [unwired: 3 in]
            n251 = local read "Heater Safety"() -> (w517:cluster{"Encl 1":bool, "Encl 2":bool})
            n252 = Unbundle(w498) -> ("data[0]"=w507:dbl, "data[1]"=w506:dbl, "data[2]"=w505:dbl)
            n253 = Boolean To (0,1)(Boolean=w517) -> (0, 1=w516:cluster{"Encl 1":i16, "Encl 2":i16})
            n254 = Cluster To Array(cluster=w516) -> (array=w515:i16[])
            n255 = To Double Precision Float(number=w515) -> (double precision float=w508:dbl[])
            n256 = local write "Room degC 1"(w505) -> ()
            n257 = local write "Room degC 2"(w505) -> ()
            n258 = local write "Encl degC 1"(w507) -> ()
            n259 = local write "Encl degC 2"(w506) -> ()
            n260 = Multiply(x=w508, y=w509) -> (x*y=w510:dbl[])
            n261 = Index Array(array=w510, index=0) -> (element=w512:dbl)
            n262 = Index Array(array=w510, index=1) -> (element=w511:dbl)
            n263 = local write "Heat% 2"(w511) -> ()
            n264 = local write "Heat% 1"(w512) -> ()
            n265 = local write "Heat%"(w510) -> ()
          }
        }
        n266 = call "Time Proportioning [array] v3.vi"("Now (mS)"=w473, "Cycle Time (mS)"=w480, "On Time (%)"=w485) -> ("Relay Output"=w490:bool[])
        n267 = flat-sequence {
          tunnel: w459 -> [w492]
          tunnel: [w492] -> w458
          tunnel: w457 -> [w491]
          frame #0 {
            n268 = Wait (ms)(milliseconds to wait=w491) -> ()  [unwired: 1 out]
          }
        }
        n269 = case shown="True" w464 {
          tunnel: w458 -> [w530 w532]
          tunnel: [w530 w531] -> w462
          tunnel: [w529 w534] -> w487
          tunnel: w486 -> [w529 _]
          tunnel: w471 -> [w528 w535]
          tunnel: [w528 w533] -> w470
          frame False {
          }
          frame True {
            n270 = call-poly "ULx Read.vi"("task in"=w535, "error in"=w532) -> ("task out"=w533:refnum<k24>, "data"=w534:bool[], "error out"=w531:errorcluster)  [unwired: 11 in]
          }
        }
        n271 = Not Equal?(x=w490, y=w489) -> (x != y?=w488:bool[])
        n272 = flat-sequence {
          tunnel: w461 -> [w494]
          tunnel: [w494] -> w460
          tunnel: w457 -> [w493]
          frame #0 {
            n273 = Wait (ms)(milliseconds to wait=w493) -> ()  [unwired: 1 out]
          }
        }
        n274 = Or Array Elements(Boolean array=w488) -> (logical OR=w465:bool)
        n275 = case shown="True" w465 {
          tunnel: w460 -> [w537 w542]
          tunnel: [w537 w541] -> w459
          tunnel: w490 -> [_ w538]
          tunnel: w469 -> [w536 w540]
          tunnel: [w536 w539] -> w468
          frame False {
          }
          frame True {
            n276 = call-poly "ULx Write.vi"("task in"=w540, "data"=w538, "error in"=w542) -> ("task out"=w539:refnum<k24>, "error out"=w541:errorcluster)  [unwired: 10 in, 1 out]
          }
        }
        n277 = Array To Cluster(array=w487) -> (cluster=w481:cluster{"data[0]":bool, "data[1]":bool})
        n278 = flat-sequence {
          tunnel: [w526] -> w484
          tunnel: w462 -> [w524]
          frame #0 {
            n279 = Unbundle By Name(w524) -> ("status"=w523:bool)
            n280 = local read "Exit 2"() -> (w525:bool)
            n281 = case shown="True" w523 {
              tunnel: w523 -> [_ w527]
              frame False {
              }
              frame True {
                n282 = property on="Exit 2" class="Bool (strict)"("Val(Sgnl)"=w527) -> ()  [unwired: 2 in, 2 out]
              }
            }
            n283 = Compound Arithmetic op=OR(w523, w525) -> (w526:bool)
          }
        }
        n284 = local write "Heater Out  T/F"(w490) -> ()
        n285 = Unbundle(w481) -> ("data[0]"=w483:bool, "data[1]"=w482:bool)
        n286 = local write "Heater Safety"(w481) -> ()
        n287 = local write "Heat Safety 1"(w483) -> ()
        n288 = local write "Heat Safety 2"(w482) -> ()
      }
      n289 = while {
        tunnel: u32 100 ("Timer loop mS") -> [w161]
        tunnel: [w154] -> w110
        tunnel: w108 -> [w157]
        tunnel: w107 -> [w156]
        tunnel: [w155] -> w106
        tunnel: w96 -> [w153]
        i -> [w159]
        stop <- w162 stop-if-true
        # "Get pressure readings using Agilent 34970A"
        n290 = local read "34970A Scan Sec"() -> (w158:u32)
        n291 = Wait Until Next ms Multiple(millisecond multiple=w161) -> ()  [unwired: 1 out]
        n292 = Equal To 0?(x=w159) -> (x = 0?=w160:bool)
        n293 = call "Interval Trigger 03.vi"("First Call?: T/F"=w160, "Iteration#"=w159, "Loop mS"=w161, "Interval Sec"=w158) -> ("Go"=w152:bool)  [unwired: 3 in, 2 out]
        n294 = case shown="True" w152 {
          tunnel: [w168 w188] -> w154
          tunnel: w157 -> [w169 w191]
          tunnel: w156 -> [w168 w189]
          tunnel: [w169 w190] -> w155
          tunnel: w153 -> [_ w187]
          frame False {
          }
          frame True {
            n295 = call "34970A Trigger+Read SW Scan v7.vi"("VISA session"=w191, "error in"=w189, "# Chan/Scan"=w187, "Error Query?"=TRUE) -> ("VISA out"=w190:refnum<visa-resource-name>, "Pressures"=w185:T5, "error"=w188:errorcluster)  [unwired: 7 in, 2 out]
            n296 = Unbundle(w185) -> ("Fill PSIA 1"=w197:dbl, "Ref PSIA 1"=w196:dbl, "Diff H2O 1"=w195:dbl, "Fill PSIA 2"=w194:dbl, "Ref PSIA 2"=w193:dbl, "Diff H2O 2"=w192:dbl)
            n297 = local read "Room degC 1"() -> (w174:dbl)
            n298 = local read "Encl degC 2"() -> (w175:dbl)
            n299 = local read "Encl degC 1"() -> (w176:dbl)
            n300 = local read "Heat% 1"() -> (w173:dbl)
            n301 = local read "Heat% 2"() -> (w172:dbl)
            n302 = Unbundle(w185) -> ("Fill PSIA 1"=w184:dbl, "Ref PSIA 1"=w183:dbl, "Diff H2O 1"=w179:dbl, "Fill PSIA 2"=w182:dbl, "Ref PSIA 2"=w181:dbl, "Diff H2O 2"=w177:dbl)
            n303 = local write "Fill PSIA 1"(w197) -> ()
            n304 = local write "Ref PSIA 1"(w196) -> ()
            n305 = local write "Diff H2O  1"(w195) -> ()
            n306 = local write "Fill PSIA 2"(w194) -> ()
            n307 = local write "Ref PSIA 2"(w193) -> ()
            n308 = local write "Diff H2O 2"(w192) -> ()
            n309 = Bundle("Fill PSIA 1"=w184, "Ref PSIA 1"=w183) -> (w180:cluster{"Fill PSIA 1":dbl, "Ref PSIA 1":dbl})  [unwired: 1 in]
            n310 = Bundle("Fill PSIA 2"=w182, "Ref PSIA 2"=w181) -> (w178:cluster{"Fill PSIA 2":dbl, "Ref PSIA 2":dbl})  [unwired: 1 in]
            n311 = Bundle("Encl degC 1"=w176, "Room degC 1"=w174) -> (w171:cluster{"Encl degC 1":dbl, "Room degC 1":dbl})  [unwired: 1 in]
            n312 = Bundle("Encl degC 2"=w175, "Room degC 1"=w174) -> (w170:cluster{"Encl degC 2":dbl, "Room degC 1":dbl})  [unwired: 1 in]
            n313 = local write "Heat% Cht 1"(w173) -> ()
            n314 = local write "Heat% Cht 2"(w172) -> ()
            n315 = local write "Absolute Pressure Cht 1"(w180) -> ()
            n316 = local write "Diff Pressure Cht 1"(w179) -> ()
            n317 = local write "Temperature Cht 1"(w171) -> ()
            n318 = local write "Temperature Cht 2"(w170) -> ()
            n319 = local write "Absolute Pressure Cht 2"(w178) -> ()
            n320 = local write "Diff Pressure Cht 2"(w177) -> ()
          }
        }
        n321 = flat-sequence {
          tunnel: [w166] -> w162
          tunnel: w154 -> [w163]
          frame #0 {
            n322 = Unbundle By Name(w163) -> ("status"=w164:bool)
            n323 = local read "Exit 2"() -> (w165:bool)
            n324 = case shown="True" w164 {
              tunnel: w164 -> [_ w167]
              frame False {
              }
              frame True {
                n325 = property on="Exit 2" class="Bool (strict)"("Val(Sgnl)"=w167) -> ()  [unwired: 2 in, 2 out]
              }
            }
            n326 = Compound Arithmetic op=OR(w164, w165) -> (w166:bool)
          }
        }
      }
      n327 = local write "Test start 1"(FALSE ("Run/Stop 1")) -> ()
      n328 = while {
        tunnel: [w125] -> w91
        shift-right: [w123] -> _
        shift-left: FALSE -> [w122]
        tunnel: w92 -> [w120]
        i -> [w119]
        stop <- w121 stop-if-true
        # "Run/Stop rising edge detector"
        # "write data from tester #1 to file"
        n329 = local read "Run/Stop 1"() -> (w123:bool)
        n330 = Greater?(x=w123, y=w122) -> (0:w124:bool)
        n331 = Wait Until Next ms Multiple(millisecond multiple=w120) -> ()  [unwired: 1 out]
        n332 = case shown="True" w123 {
          tunnel: [errorcluster {"status"=FALSE, "code"=0, "source"=""} ("error out") w134] -> w125
          tunnel: w119 -> [_ w128]
          tunnel: w124 -> [_ w132]
          tunnel: w120 -> [_ w133]
          frame False {
          }
          frame True {
            n333 = local read "File Log Sec"() -> (w131:u32)
            n334 = call "Interval Trigger 03.vi"("First Call?: T/F"=w132, "Iteration#"=w128, "Loop mS"=w133, "Interval Sec"=w131) -> ("Go"=w130:bool, "Timestamp sec"=w129:u32)  [unwired: 3 in, 1 out]
            n335 = case shown="True" w130 {
              tunnel: [errorcluster {"status"=FALSE, "code"=0, "source"=""} ("error out") w149] -> w134
              tunnel: w129 -> [_ w144]
              frame False {
              }
              frame True {
                n336 = local read "Diff H2O  1"() -> (w136:dbl)
                n337 = local read "Fill PSIA 1"() -> (w138:dbl)
                n338 = local read "Ref PSIA 1"() -> (w137:dbl)
                n339 = local read "Encl degC 1"() -> (w140:dbl)
                n340 = local read "Room degC 1"() -> (w139:dbl)
                n341 = local read "Heat% 1"() -> (w141:dbl)
                n342 = local read "Fallback Location"() -> (w142:T2)
                n343 = local read "Log Dir Path"() -> (w143:path)
                n344 = local read "Time Fmt"() -> (w146:enum16{"H:M:S", "Days", "Secs"})
                n345 = local read "Filename 1"() -> (w150:string)
                n346 = local read "Header"() -> (w148:string[])
                n347 = Bundle("Fill PSIA 1"=w138, "Ref PSIA 1"=w137, "Diff H2O  1"=w136, "Encl degC 1"=w140, "Room degC 1"=w139, "Heat% 1"=w141) -> (w145:T15)  [unwired: 1 in]
                n348 = call "Leaktest Data to File v10.vi"("Elapsed Sec"=w144, "Dir Path"=w143, "Fallback Location"=w142, "File Name"=w150, "Time Fmt"=w146, "Leaktest Data"=w145, "Header"=w148, "Tester"="Tester1") -> ("error out"=w149:errorcluster)  [unwired: 7 in]
                n349 = case shown="Error" w149 {
                  frame No Error {
                  }
                  frame Error {
                    n350 = One Button Dialog(message="Tester 1 cannot write to the data file. Clear the problem and continue.") -> ()  [unwired: 1 in, 1 out]
                  }
                }
              }
            }
          }
        }
        n351 = flat-sequence {
          tunnel: [w126] -> w121
          frame #0 {
            n352 = local read "Exit 2"() -> (w126:bool)
          }
        }
      }
      n353 = while {
        tunnel: [w204] -> w98
        shift-right: [w202] -> _
        shift-left: FALSE -> [w201]
        tunnel: w92 -> [w199]
        i -> [w198]
        stop <- w200 stop-if-true
        # "Run/Stop rising edge detector"
        # "write data from tester #2 to file"
        n354 = local read "Run/Stop 2"() -> (w202:bool)
        n355 = Greater?(x=w202, y=w201) -> (0:w203:bool)
        n356 = Wait Until Next ms Multiple(millisecond multiple=w199) -> ()  [unwired: 1 out]
        n357 = case shown="True" w202 {
          tunnel: [errorcluster {"status"=FALSE, "code"=0, "source"=""} ("error out") w213] -> w204
          tunnel: w198 -> [_ w207]
          tunnel: w203 -> [_ w211]
          tunnel: w199 -> [_ w212]
          frame False {
          }
          frame True {
            n358 = local read "File Log Sec"() -> (w210:u32)
            n359 = call "Interval Trigger 03.vi"("First Call?: T/F"=w211, "Iteration#"=w207, "Loop mS"=w212, "Interval Sec"=w210) -> ("Go"=w209:bool, "Timestamp sec"=w208:u32)  [unwired: 3 in, 1 out]
            n360 = case shown="True" w209 {
              tunnel: [errorcluster {"status"=FALSE, "code"=0, "source"=""} ("error out") w228] -> w213
              tunnel: w208 -> [_ w223]
              frame False {
              }
              frame True {
                n361 = local read "Fill PSIA 2"() -> (w217:dbl)
                n362 = local read "Ref PSIA 2"() -> (w216:dbl)
                n363 = local read "Diff H2O 2"() -> (w215:dbl)
                n364 = local read "Encl degC 2"() -> (w219:dbl)
                n365 = local read "Room degC 2"() -> (w218:dbl)
                n366 = local read "Heat% 2"() -> (w220:dbl)
                n367 = local read "Fallback Location"() -> (w221:T2)
                n368 = local read "Log Dir Path"() -> (w222:path)
                n369 = local read "Time Fmt"() -> (w225:enum16{"H:M:S", "Days", "Secs"})
                n370 = local read "Filename 2"() -> (w229:string)
                n371 = local read "Header"() -> (w227:string[])
                n372 = Bundle("Fill PSIA 2"=w217, "Ref PSIA 2"=w216, "Diff H2O 2"=w215, "Encl degC 2"=w219, "Room degC 2"=w218, "Heat% 2"=w220) -> (w224:T16)  [unwired: 1 in]
                n373 = call "Leaktest Data to File v10.vi"("Elapsed Sec"=w223, "Dir Path"=w222, "Fallback Location"=w221, "File Name"=w229, "Time Fmt"=w225, "Leaktest Data"=w224, "Header"=w227, "Tester"="Tester2") -> ("error out"=w228:errorcluster)  [unwired: 7 in]
                n374 = case shown="Error" w228 {
                  frame No Error {
                  }
                  frame Error {
                    n375 = One Button Dialog(message="Tester 2 cannot write to the data file. Clear the problem and continue.") -> ()  [unwired: 1 in, 1 out]
                  }
                }
              }
            }
          }
        }
        n376 = flat-sequence {
          tunnel: [w205] -> w200
          frame #0 {
            n377 = local read "Exit 2"() -> (w205:bool)
          }
        }
      }
      n378 = Merge Errors(w91, w98, w97, w90, w110) -> (w88:errorcluster)
    }
    frame Error {
    }
  }
  n379 = flat-sequence {
    tunnel: w38 -> [w555]
    frame #0 {
      w561 = T12."Disabled and Grayed Out" ("Disabled")
      w560 = T12."Enabled" ("Disabled")
      n380 = control-ref of="Test start 2"() -> (w557:refnum<vi>)
      n381 = control-ref of="Test start 1"() -> (w556:refnum<vi>)
      n382 = control-ref of="Test stop 1"() -> (w558:refnum<vi>)
      n383 = control-ref of="Test stop 2"() -> (w559:refnum<vi>)
      n384 = local write "Control Mode"(cluster{"Encl 1":T9, "Encl 2":T9} {"Encl 1"=enum."Off", "Encl 2"=enum."Off"} ("Control Mode")) -> ()
      n385 = local write "Run/Stop 1"(FALSE ("Run/Stop 1")) -> ()
      n386 = local write "Run/Stop 2"(FALSE ("Run/Stop 1")) -> ()
      n387 = property class="Bool (strict)"(reference=w556, "DisabledEnum"=w560, "Value"=w555) -> ()  [unwired: 1 in, 2 out]
      n388 = property class="Bool (strict)"(reference=w557, "DisabledEnum"=w560, "Value"=w555) -> ()  [unwired: 1 in, 2 out]
      n389 = property class="Bool (strict)"(reference=w558, "DisabledEnum"=w561, "Value"=w555) -> ()  [unwired: 1 in, 2 out]
      n390 = property class="Bool (strict)"(reference=w559, "DisabledEnum"=w561, "Value"=w555) -> ()  [unwired: 1 in, 2 out]
      n391 = local write "Run/Stop 1"(w555) -> ()
      n392 = local write "Run/Stop 2"(w555) -> ()
    }
  }
  n393 = Unbundle(w42) -> ("Encl 1"=w43:bool, "Encl 2"=w44:bool)
  n394 = local write "Heater Safety"(w42) -> ()
  n395 = local write "Exit"(w39) -> ()
  n396 = local write "Exit 2"(w39) -> ()
  n397 = local write "Heater Out  T/F"(w1) -> ()
  n398 = local write "Heat Safety 1"(w43) -> ()
  n399 = local write "Heat Safety 2"(w44) -> ()
  n400 = call "HP34970A Trigger.vi"("Command (0:Rem Trig)"=T11."Abort Scan" ("Command"), "VISA session"=w13) -> ("dup VISA session"=w16:refnum<visa-resource-name>)  [unwired: 7 in, 1 out]
  n401 = call "34970 Error Query (Multiple)+++.vi"("VISA resource name"=w16, "error in (no error)"=w14) -> ("VISA resource name out"=w15:refnum<visa-resource-name>, "error out"=w18:errorcluster)  [unwired: 10 in, 2 out]
  n402 = VISA Close(VISA resource name=w15, error in (no error)=w18) -> (error out=w8:errorcluster)
  n403 = call "ULx Clear Task.vi"("task in"=w9, "error in"=w8) -> ("error out"=w7:errorcluster)  [unwired: 13 in]
  n404 = call-poly "ULx Write.vi"("task in"=w5, "data"=w1, "error in"=w7) -> ("task out"=w10:refnum<k24>, "error out"=w11:errorcluster)  [unwired: 10 in, 1 out]
  n405 = call "ULx Clear Task.vi"("task in"=w10, "error in"=w11) -> ("error out"=w2:errorcluster)  [unwired: 13 in]
  "error out" <- w2
  n406 = call "ULx Clear Task.vi"("task in"=w3, "error in"=w2) -> ()  [unwired: 13 in, 1 out]
  n407 = call "Simple Error Handler.vi"("error in (no error)"=w2) -> ()  [unwired: 4 in, 5 out]
